vi "LVFunction_Imop_SlopesPostProcessor_Apply Pupil.vi"(0 "HasoSlopes in":refnum<class "HasoSlopes.lvclass">, 5 "HasoSlopes OUT":refnum<class "HasoSlopes.lvclass">, 7 "Pupil IN":refnum<class "Pupil.lvclass">, 11 "error in (no error)":errorcluster) -> (4 "HasoSlopes out":refnum<class "HasoSlopes.lvclass">, 6 "HasoSlopes OUT 2":refnum<class "HasoSlopes.lvclass">, 15 "error out":errorcluster)   [LabVIEW 2020]
uses:
  HasoSlopes.lvclass
  Pupil.lvclass
  LVClass_HasoSlopes Read HasoSlopes _ property.vi
  LVClass_Pupil Read Pupil.vi
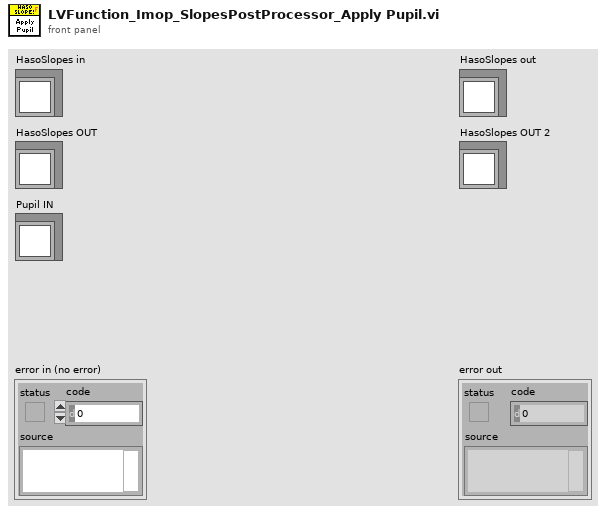
[diagram p1: front panel]
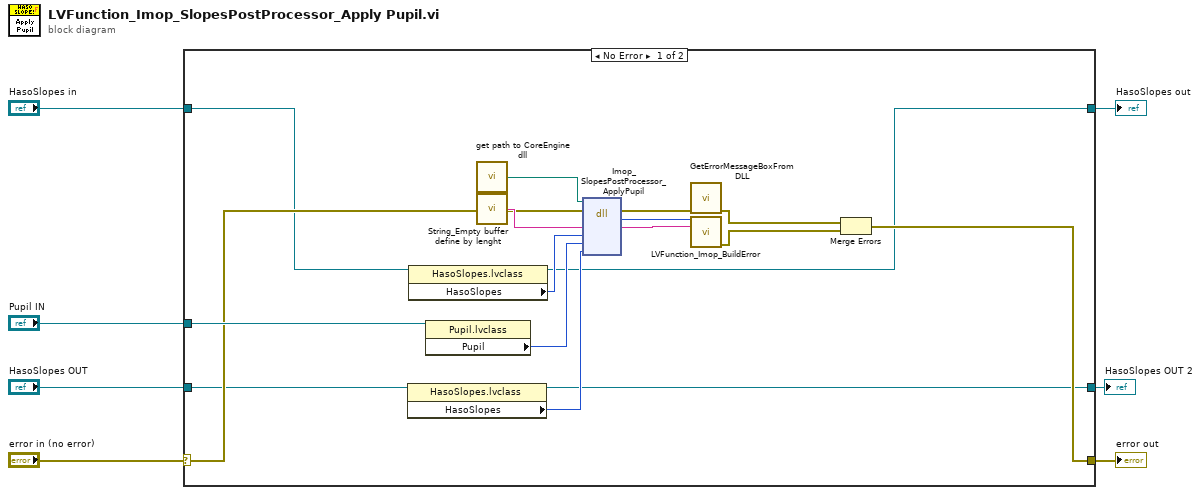
[diagram p0: block diagram]
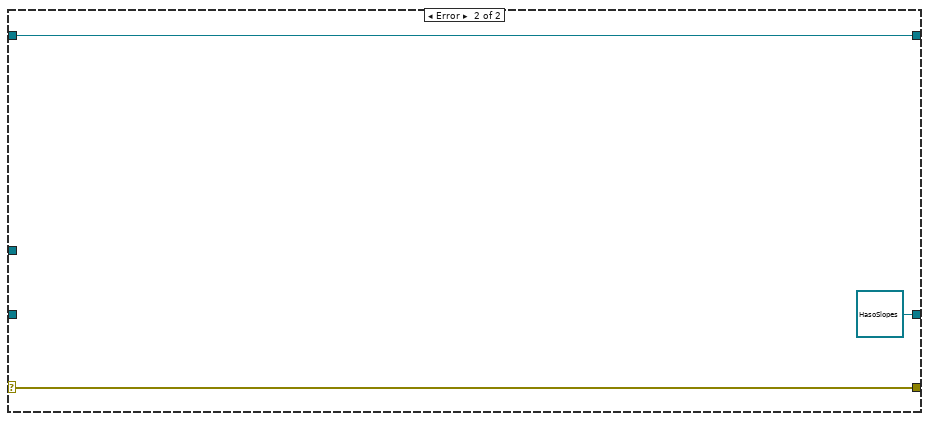
[diagram p2: hidden frame]
diagram:
  n1 = case shown="No Error" "error in (no error)" {
    selector: "error in (no error)" -> [w14 w27]
    tunnel: [w13 w27] -> w6
    tunnel: [w8 w26] -> w4
    tunnel: "HasoSlopes in" -> [w9 w26]
    tunnel: "Pupil IN" -> [w15 _]
    tunnel: "HasoSlopes OUT" -> [w12 _]
    tunnel: [w10 refnum<class "HasoSlopes.lvclass"> refnum ("HasoSlopes OUT")] -> w1
    frame No Error {
      n2 = property class="HasoSlopes.lvclass"(reference=w12) -> (reference out=w10:refnum<class "HasoSlopes.lvclass">, "HasoSlopes"=w11:i32)  [unwired: 1 in, 1 out]
      n3 = property class="HasoSlopes.lvclass"(reference=w9) -> (reference out=w8:refnum<class "HasoSlopes.lvclass">, "HasoSlopes"=w23:i32)  [unwired: 1 in, 1 out]
      n4 = property class="Pupil.lvclass"(reference=w15) -> ("Pupil"=w24:i32)  [unwired: 1 in, 2 out]
      n5 = call "get path to CoreEngine dll.vi"() -> ("path to c_interface_vc100.dll"=w18:path)  [unwired: 12 in, 3 out]
      n6 = call "String_Empty buffer define by lenght.vi"() -> ("Empty buffer"=w19:string)  [unwired: 1 in]
      n7 = dll-call lib="D:/FLE/0.Code/CoreEngine4_Suite/LV2011_interface/DLLs/c_interface_vc100.dll" fn="Imop_SlopesPostProcessor_ApplyPupil"(path in=w18, error in=w14, "Message"=w19, "HasoSlopes IN"=w23, "Pupil"=w24, "HasoSlopes OUT"=w11) -> (error out=w22:errorcluster, "return type"=w20:i32, "Message"=w21:string)  [unwired: 4 in, 1 out]
      n8 = call "GetErrorMessageBoxFromDLL.vi"("error IN"=w22) -> ("error OUT"=w17:errorcluster)  [unwired: 10 in]
      n9 = call "LVFunction_Imop_BuildError.vi"("code"=w20, "String to Prepend to source (\"\")"=w21) -> ("error out"=w16:errorcluster)  [unwired: 13 in]
      n10 = Merge Errors(w17, w16) -> (w13:errorcluster)
    }
    frame Error {
    }
  }
  "error out" <- w6
  "HasoSlopes out" <- w4
  "HasoSlopes OUT 2" <- w1
